vi "settings.vi"(8 "Error In":errorcluster) -> (0 "Error Out":errorcluster)   [LabVIEW 2012]
uses:
  Scanning Setting.vi
panel:
  in  "Z-Thickness":dbl(slide)=0.15 scale=0.0..0.3
  in  "Ofset":dbl=410.64
  in  "Location       =DxZ-Pluse    +":dbl=482.42
  in  "B":dbl=9.46
  in  "Peizo Voltage=MxZ-Pluse    +":dbl=11.35
  out "Calibration Table":string[][](table)
  in  "Peizo":dbl=6.0
  in  "Z-Plus":dbl(slide)=-0.45 step=0.01 scale=0.0..-0.7
  in  "1000Hz":bool
  in  "30fps":bool
  in  "100fps":bool
  in  "Single line Scan":bool
  in  "Default":bool
  in  "S Angle Correction (ratio)":dbl(knob)=-0.29473162999791414 scale=-0.5..0.5
  in  "Z-offset":dbl(slide)=-1.0299401197604787 scale=-4.0..4.0
  in  "Cancel Button":bool
  in  "OK Button":bool
  in  "S-offset":dbl(slide)=-2.175438596491228 scale=-4.0..4.0
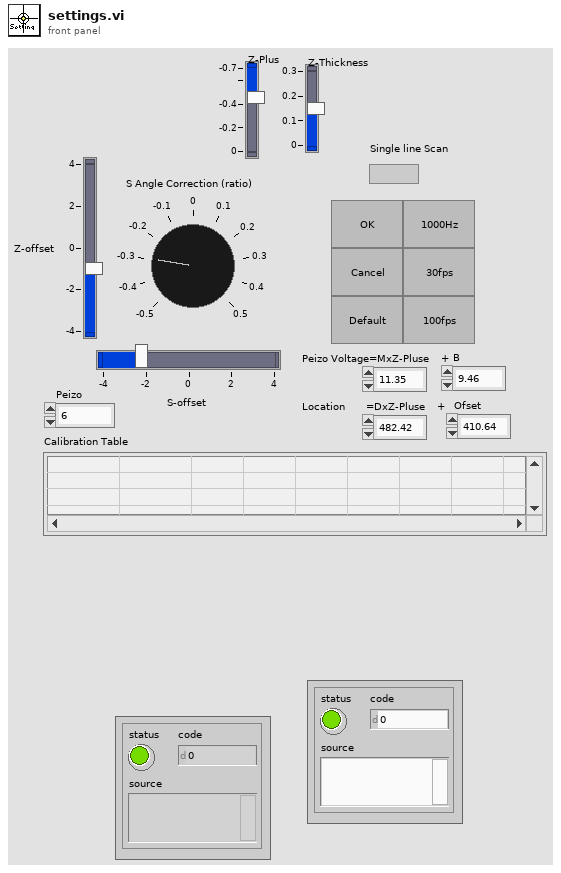
[diagram p1: front panel]
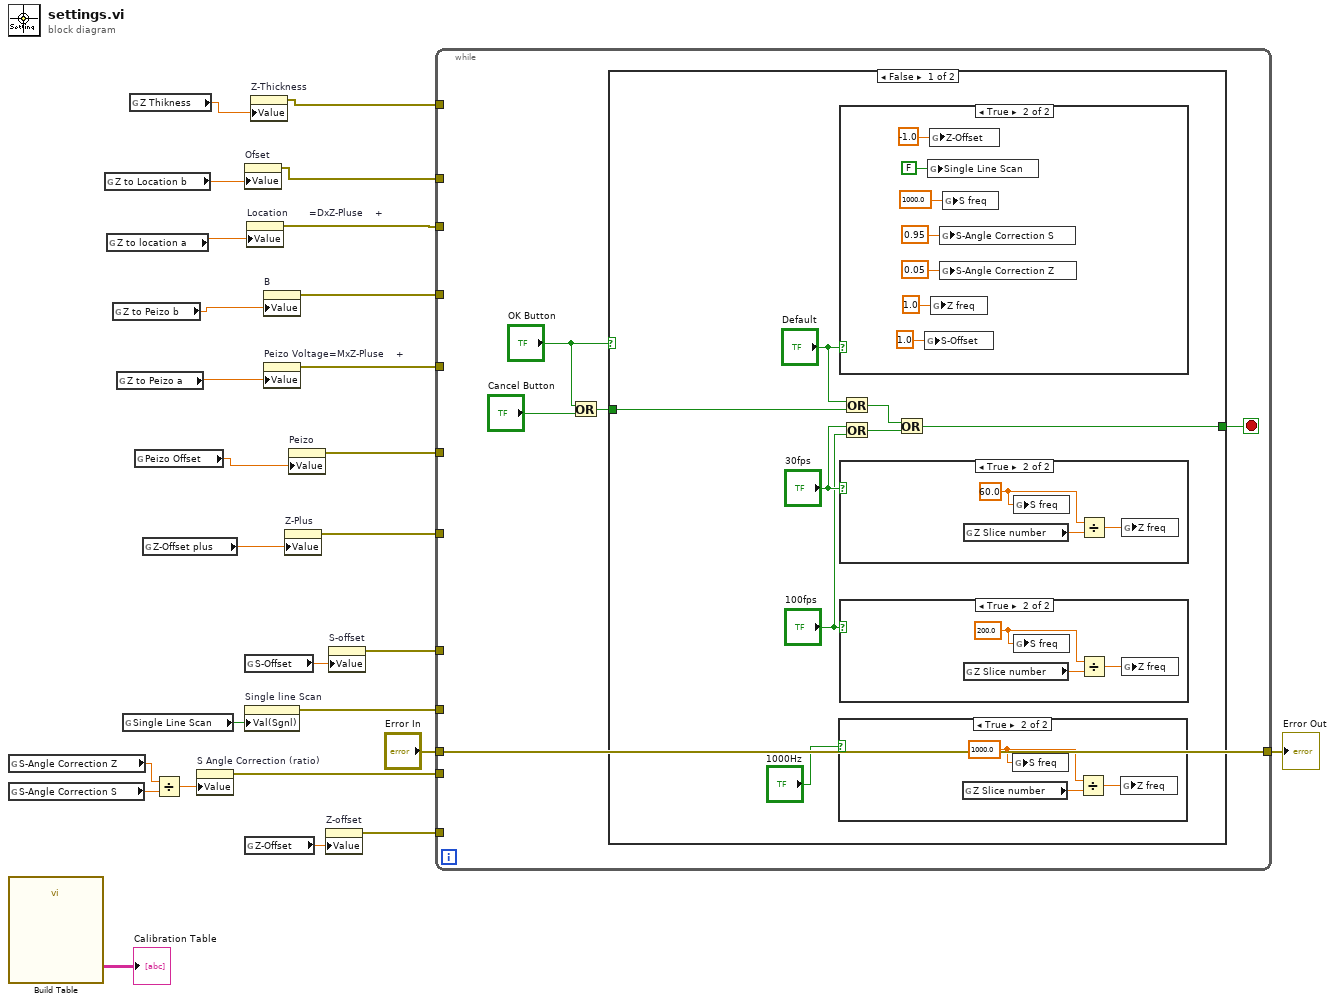
[diagram p0: block diagram]
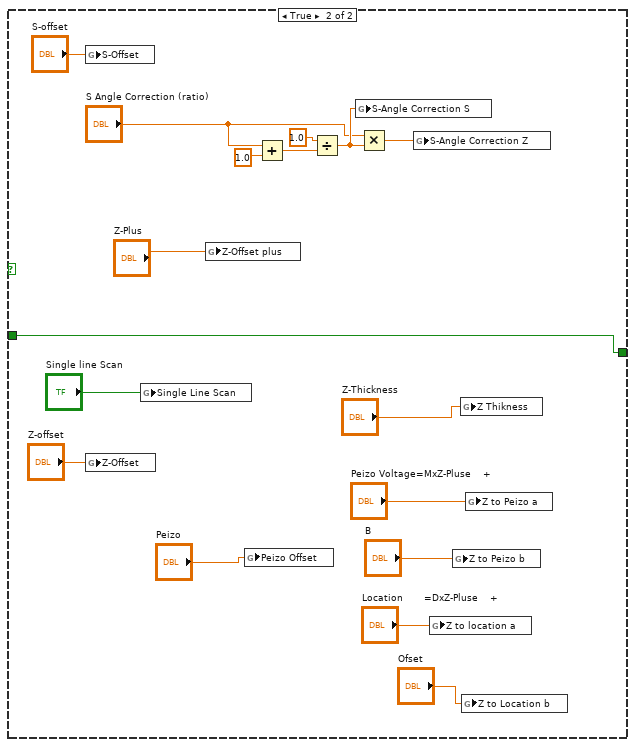
[diagram p6: hidden frame]
diagram:
  n1 = global read "Scanning Setting.vi" "S-Angle Correction Z"() -> (w21:dbl)
  n2 = global read "Scanning Setting.vi" "S-Angle Correction S"() -> (w20:dbl)
  n3 = call "Build Table"() -> ("Table"=→"Calibration Table":string[][])  [unwired: 5 in, 6 out]
  n4 = global read "Scanning Setting.vi" "Z to Location b"() -> (w4:dbl)
  n5 = global read "Scanning Setting.vi" "Z to location a"() -> (w6:dbl)
  n6 = global read "Scanning Setting.vi" "Z to Peizo b"() -> (w8:dbl)
  n7 = global read "Scanning Setting.vi" "Z to Peizo a"() -> (w10:dbl)
  n8 = global read "Scanning Setting.vi" "Single Line Scan"() -> (w17:bool)
  n9 = global read "Scanning Setting.vi" "Z Thikness"() -> (w2:dbl)
  n10 = global read "Scanning Setting.vi" "Peizo Offset"() -> (w13:dbl)
  n11 = global read "Scanning Setting.vi" "Z-Offset plus"() -> (w15:dbl)
  n12 = Divide(x=w21, y=w20) -> (x/y=w19:dbl)
  n13 = property on="S Angle Correction (ratio)" class="Knob (strict)"("Value"=w19) -> (error out=w18:errorcluster)  [unwired: 2 in, 1 out]
  n14 = property on="Ofset" class="DigNum (strict)"("Value"=w4) -> (error out=w3:errorcluster)  [unwired: 2 in, 1 out]
  n15 = global read "Scanning Setting.vi" "S-Offset"() -> (w27:dbl)
  n16 = property on="Single line Scan" class="Bool (strict)"("Val(Sgnl)"=w17) -> (error out=w16:errorcluster)  [unwired: 2 in, 1 out]
  n17 = global read "Scanning Setting.vi" "Z-Offset"() -> (w25:dbl)
  n18 = property on="Location       =DxZ-Pluse    +" class="DigNum (strict)"("Value"=w6) -> (error out=w5:errorcluster)  [unwired: 2 in, 1 out]
  n19 = property on="Z-Thickness" class="Slide (strict)"("Value"=w2) -> (error out=w1:errorcluster)  [unwired: 2 in, 1 out]
  n20 = property on="B" class="DigNum (strict)"("Value"=w8) -> (error out=w7:errorcluster)  [unwired: 2 in, 1 out]
  n21 = property on="Peizo Voltage=MxZ-Pluse    +" class="DigNum (strict)"("Value"=w10) -> (error out=w9:errorcluster)  [unwired: 2 in, 1 out]
  n22 = property on="Z-Plus" class="Slide (strict)"("Value"=w15) -> (error out=w14:errorcluster)  [unwired: 2 in, 1 out]
  n23 = property on="Peizo" class="DigNum (strict)"("Value"=w13) -> (error out=w12:errorcluster)  [unwired: 2 in, 1 out]
  n24 = property on="Z-offset" class="Slide (strict)"("Value"=w25) -> (error out=w24:errorcluster)  [unwired: 2 in, 1 out]
  n25 = property on="S-offset" class="Slide (strict)"("Value"=w27) -> (error out=w26:errorcluster)  [unwired: 2 in, 1 out]
  n26 = while {
    tunnel: w26 -> [_]
    tunnel: w24 -> [_]
    tunnel: "Error In" -> [w28]
    tunnel: [w28] -> w22
    tunnel: w18 -> [_]
    tunnel: w16 -> [_]
    tunnel: w14 -> [_]
    tunnel: w12 -> [_]
    tunnel: w9 -> [_]
    tunnel: w7 -> [_]
    tunnel: w5 -> [_]
    tunnel: w3 -> [_]
    tunnel: w1 -> [_]
    stop <- w29 stop-if-true
    n27 = Or(x="OK Button", y="Cancel Button") -> (x .or. y?=w30:bool)
    n28 = case shown="False" "OK Button" {
      tunnel: w30 -> [w39 w72]
      tunnel: [w34 w72] -> w29
      frame False {
        n29 = case shown="True" "1000Hz" {
          frame False {
          }
          frame True {
            w43 = 1000.0 ("S freq")
            n30 = global read "Scanning Setting.vi" "Z Slice number"() -> (w42:dbl)
            n31 = global write "Scanning Setting.vi" "S freq"(w43) -> ()
            n32 = Divide(x=w43, y=w42) -> (x/y=w41:dbl)
            n33 = global write "Scanning Setting.vi" "Z freq"(w41) -> ()
          }
        }
        n34 = case shown="True" "Default" {
          frame False {
          }
          frame True {
            n35 = global write "Scanning Setting.vi" "S-Offset"(1.0 ("S-Offset")) -> ()
            n36 = global write "Scanning Setting.vi" "Single Line Scan"(FALSE ("Single Line Scan")) -> ()
            n37 = global write "Scanning Setting.vi" "Z-Offset"(-1.0 ("Z-Offset")) -> ()
            n38 = global write "Scanning Setting.vi" "Z freq"(1.0 ("Z freq")) -> ()
            n39 = global write "Scanning Setting.vi" "S-Angle Correction S"(0.95 ("S-Angle Correction S")) -> ()
            n40 = global write "Scanning Setting.vi" "S-Angle Correction Z"(0.05 ("S-Angle Correction Z")) -> ()
            n41 = global write "Scanning Setting.vi" "S freq"(1000.0 ("S freq")) -> ()
          }
        }
        n42 = case shown="True" "30fps" {
          frame False {
          }
          frame True {
            w49 = 60.0 ("S freq")
            n43 = global read "Scanning Setting.vi" "Z Slice number"() -> (w48:dbl)
            n44 = global write "Scanning Setting.vi" "S freq"(w49) -> ()
            n45 = Divide(x=w49, y=w48) -> (x/y=w47:dbl)
            n46 = global write "Scanning Setting.vi" "Z freq"(w47) -> ()
          }
        }
        n47 = case shown="True" "100fps" {
          frame False {
          }
          frame True {
            w46 = 200.0 ("S freq")
            n48 = global read "Scanning Setting.vi" "Z Slice number"() -> (w45:dbl)
            n49 = global write "Scanning Setting.vi" "S freq"(w46) -> ()
            n50 = Divide(x=w46, y=w45) -> (x/y=w44:dbl)
            n51 = global write "Scanning Setting.vi" "Z freq"(w44) -> ()
          }
        }
        n52 = Or(x="Default", y=w39) -> (x .or. y?=w35:bool)
        n53 = Or(x="30fps", y="100fps") -> (x .or. y?=w36:bool)
        n54 = Or(x=w35, y=w36) -> (x .or. y?=w34:bool)
      }
      frame True {
        n55 = global write "Scanning Setting.vi" "S-Offset"("S-offset") -> ()
        n56 = global write "Scanning Setting.vi" "Z-Offset"("Z-offset") -> ()
        n57 = global write "Scanning Setting.vi" "Single Line Scan"("Single line Scan") -> ()
        n58 = global write "Scanning Setting.vi" "Z-Offset plus"("Z-Plus") -> ()
        n59 = global write "Scanning Setting.vi" "Peizo Offset"("Peizo") -> ()
        n60 = Add(x="S Angle Correction (ratio)", y=1.0) -> (x+y=w69:dbl)
        n61 = Divide(x=1.0, y=w69) -> (x/y=w67:dbl)
        n62 = global write "Scanning Setting.vi" "S-Angle Correction S"(w67) -> ()
        n63 = Multiply(x="S Angle Correction (ratio)", y=w67) -> (x*y=w65:dbl)
        n64 = global write "Scanning Setting.vi" "S-Angle Correction Z"(w65) -> ()
        n65 = global write "Scanning Setting.vi" "Z to location a"("Location       =DxZ-Pluse    +") -> ()
        n66 = global write "Scanning Setting.vi" "Z to Peizo b"("B") -> ()
        n67 = global write "Scanning Setting.vi" "Z Thikness"("Z-Thickness") -> ()
        n68 = global write "Scanning Setting.vi" "Z to Location b"("Ofset") -> ()
        n69 = global write "Scanning Setting.vi" "Z to Peizo a"("Peizo Voltage=MxZ-Pluse    +") -> ()
      }
    }
  }
  "Error Out" <- w22
